vi "Start.vi"(8 "error in (no error)":errorcluster, 11 "Framework in":refnum<class "Framework.lvclass">) -> (0 "error out":errorcluster, 3 "Framework out":refnum<class "Framework.lvclass">)   [LabVIEW 2017, in "DSF Core.lvlib" / "Framework.lvclass"]
uses:
  Framework.lvclass
  Plugin/Plugin.lvclass
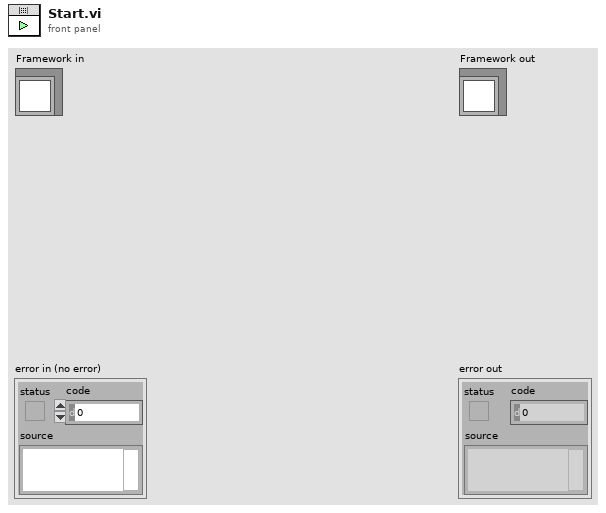
[diagram p1: front panel]
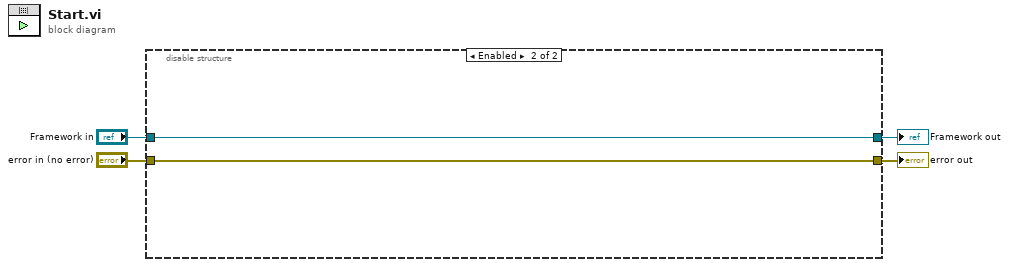
[diagram p0: block diagram]
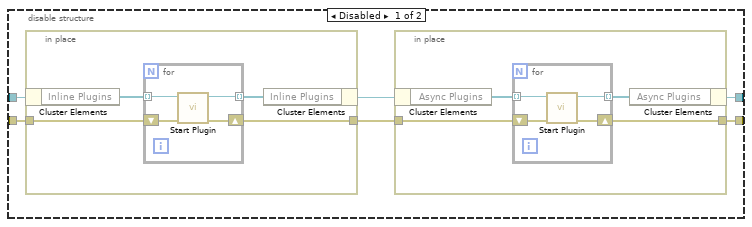
[diagram p2: hidden frame]
diagram:
  n1 = disable-structure shown="Enabled" {
    disable-tunnel: [w10 w27] -> w4
    disable-tunnel: [w9 w28] -> w3
    disable-tunnel: "Framework in" -> [w8 w28]
    disable-tunnel: "error in (no error)" -> [w7 w27]
    frame Disabled {
      n2 = in-place {
        in-place-border: w7 -> [w11]
        in-place-border: [w14] -> w6
        n3 = in-place-cluster #1(w8) -> ("Inline Plugins"=w13:refnum<class "Plugin.lvclass">[])
        n4 = for {
          tunnel: w13 -> [w18] mode=indexing
          tunnel: [w17] -> w12 mode=indexing
          shift-right: [w16] -> w14
          shift-left: w11 -> [w15]
          n5 = call "Start Plugin.vi"("error in (no error)"=w15, "Plugin in"=w18) -> ("error out"=w16:errorcluster, "Plugin out"=w17:refnum<class "Plugin.lvclass">)  [unwired: 8 in]
        }
        n6 = in-place-cluster #1("Inline Plugins"=w12) -> (w5:refnum<class "Framework.lvclass">)
      }
      n7 = in-place {
        in-place-border: w6 -> [w19]
        in-place-border: [w22] -> w10
        n8 = in-place-cluster #2(w5) -> ("Async Plugins"=w21:refnum<class "Plugin.lvclass">[])
        n9 = for {
          tunnel: w21 -> [w26] mode=indexing
          tunnel: [w25] -> w20 mode=indexing
          shift-right: [w24] -> w22
          shift-left: w19 -> [w23]
          n10 = call "Start Plugin.vi"("error in (no error)"=w23, "Plugin in"=w26) -> ("error out"=w24:errorcluster, "Plugin out"=w25:refnum<class "Plugin.lvclass">)  [unwired: 8 in]
        }
        n11 = in-place-cluster #2("Async Plugins"=w20) -> (w9:refnum<class "Framework.lvclass">)
      }
    }
    frame Enabled {
    }
  }
  "error out" <- w4
  "Framework out" <- w3
